vi "Create Error To Be Logged.vi"(1 "Error Type":T1, 2 "Handled Error":T3) -> (0 "Error to be logged to file":T2)   [LabVIEW 2016, in "Error Manager.lvlib"]
doc: "Blank VI with error handling."
uses:
  Error Manager.lvlib
  Error Log/Error Type (enum).ctl
  Error Log/Error Log.lvclass
  Error Log/Error to be logged (cluster).ctl
  Read-Unread Status (enum).ctl
  Handled Error (cluster).ctl
panel:
  # "Input\nInputs to the VI"
  # "Development\nControls or indicators that are useful for development or testing, but which are not outputs of the VI."
  # "Output\nOutputs of the VI"
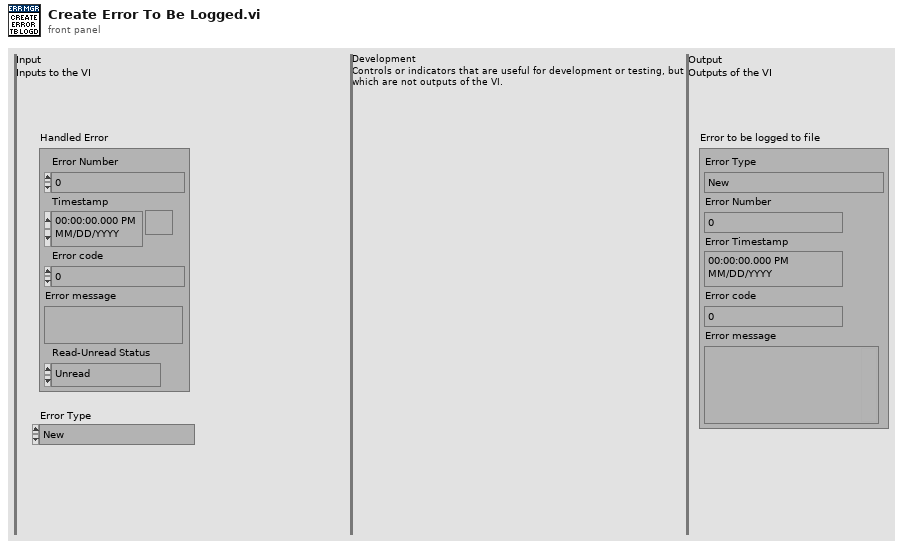
[diagram p1: front panel]
types:
  T1 = typedef "Error Manager.lvlib/Error Log.lvclass/Error Type (enum).ctl" = enum16{"New", "Identical to last logged error"}
  T2 = typedef "Error Manager.lvlib/Error Log.lvclass/Error to be logged (cluster).ctl" = cluster{"Error Type":T1, "Error Number":i32, "Error Timestamp":timestamp, "Error code":i32, "Error message":string}
  T3 = typedef "Error Manager.lvlib/Handled Error (cluster).ctl" = cluster{"Error Number":i32, "Timestamp":timestamp, "Error code":i32, "Error message":string, "Read-Unread Status":T4}
  T4 = typedef "Error Manager.lvlib/Read-Unread Status (enum).ctl" = enum16{"Unread", "Read"}
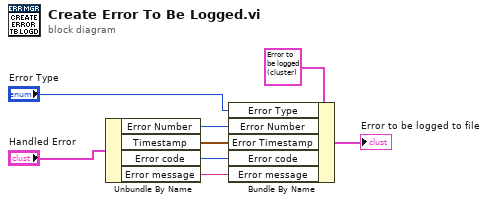
[diagram p0: block diagram]
diagram:
  n1 = Unbundle By Name("Handled Error") -> ("Error Number"=w1:i32, "Timestamp"=w5:timestamp, "Error code"=w4:i32, "Error message"=w3:string)
  n2 = Bundle By Name(cluster=T2 {"Error Type"=enum."New", "Error Number"=0, "Error Timestamp"=timestamp(0 s since 1904-01-01), "Error code"=0, "Error message"=""} ("Error to be logged"), "Error Type"="Error Type", "Error Number"=w1, "Error Timestamp"=w5, "Error code"=w4, "Error message"=w3) -> (→"Error to be logged to file":T2)
